vi "Save_Destination_Type.vi"(8 "error in (no error)":errorcluster, 9 "index":i32, 10 "buildObject":T1, 11 "AB_Dest_LLB in":refnum<class "AB_Dest_LLB.lvclass">) -> (0 "error out":errorcluster, 3 "AB_Dest_LLB out":refnum<class "AB_Dest_LLB.lvclass">)   [LabVIEW 2020, in "AB_Dest_LLB.lvclass"]
uses:
  <vilib>/AppBuilder/AB_Classes/Destination/Dest_LLB/AB_Dest_LLB.lvclass
  <resource>/Framework/Providers/API/ItemRef.ctl
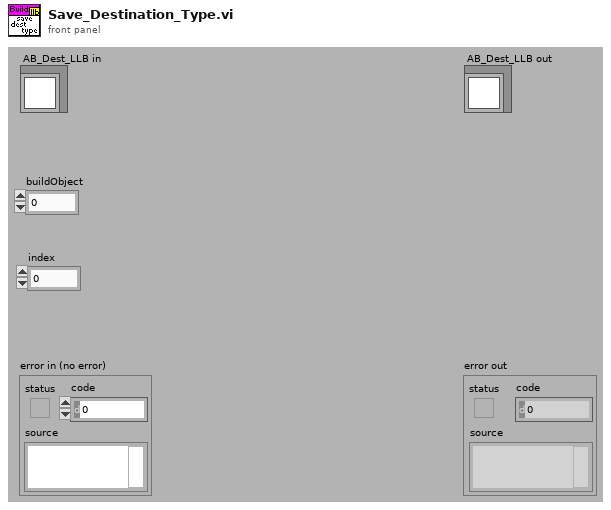
[diagram p1: front panel]
types:
  T1 = typedef "ItemRef.ctl" = u64
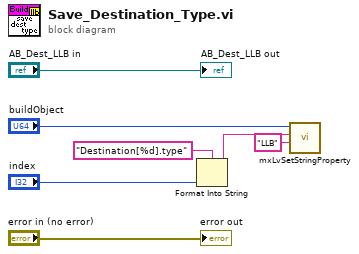
[diagram p0: block diagram]
diagram:
  n1 = Format Into String(format string="Destination[%d].type", "index") -> (resulting string=w4:string)  [unwired: 2 in, 1 out]
  n2 = call <resource>:"mxLvSetStringProperty.vi"("Value (\"\")"="LLB" ("Value (\"\")"), "Tag"=w4, "Item"="buildObject") -> ()  [unwired: 7 in, 2 out]
  "error out" <- "error in (no error)"
  "AB_Dest_LLB out" <- "AB_Dest_LLB in"
